vi "FPGA_encoder.vi"(3 "Encoder Channel B":refnum<k21>="ConnectorB/DIO1", 4 "Encoder Channel A":refnum<k21>="ConnectorB/DIO1", 5 "Velocity Interval (uSec)":u32=1000, 6 "Position Reset":bool) -> (0 "Velocity (Counts/Interval)":i32, 1 "Acceleration (Counts/Interval)":i32, 2 "Position (Counts)":i32)   [LabVIEW 2019]
doc: "This is an FPGA vi for Quadrature Encoder Velocity and Acceleration Estimation using CompactRIO. It requires as inputs a Fixed Time Interval for velocity and acceleration estimation.\n\nThis application is designed to work with an R-Series expansion setup using PCI/PXI-7811R FPGA device and a CompactRIO cRIO-9411 digital input module installed in slot 1 of the expansion chassis."
uses:
  <vilib>/rvi/Emulation/niFpgaGetClockAttributes.vi
  <vilib>/rvi/Emulation/niFpgaSctlEmulationGetInTimedLoop.vi
  <vilib>/rvi/Emulation/niFpgaEmulationReportErrorSimple.vi
  <vilib>/rvi/eio/common/nirviEmuTemplateMethod_errors.vi
  <vilib>/rvi/Emulation/niFpgaCriticalErrorInLSC.vi
  <vilib>/eio/EIONode/EIONode.xnode
  <vilib>/rvi/Arithmetic/AddSubMult/XNode/nirviSatArithmetic.xnode
panel:
  # "FPGA Application for Quadrature Encoder Velocity and \nAcceleration Estimation using CompactRIO.\n\nThis application is designed to work with an R-Series expansion setup \nusing FPGA-7811R and a CompactRIO cRIO-9411 digital input module \ninstalled in slot 1 of the expansion chassis."
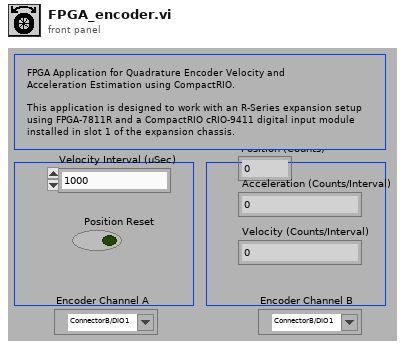
[diagram p1: front panel]
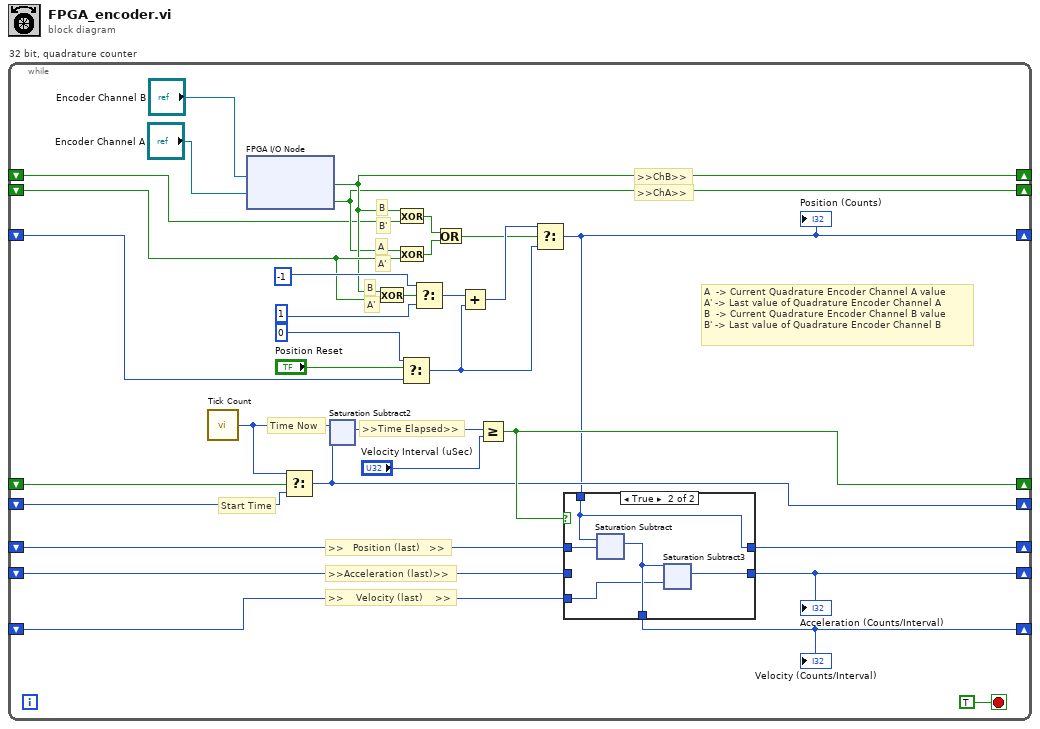
[diagram p0: block diagram]
diagram:
  n1 = while "32 bit, quadrature counter" {
    shift-right: [w22] -> _
    shift-left: _ -> [w8]
    shift-right: [w7] -> _
    shift-left: _ -> [w19]
    shift-right: [w21] -> _
    shift-left: _ -> [w23]
    shift-right: [w15] -> _
    shift-left: _ -> [w18]
    shift-right: [w10] -> _
    shift-left: _ -> [w16]
    shift-right: [w4] -> _
    shift-left: _ -> [w13]
    shift-right: [w5] -> _
    shift-left: _ -> [w12]
    shift-right: [w6] -> _
    shift-left: _ -> [w9]
    stop <- TRUE stop-if-true
    # "A  -> Current Quadrature Encoder Channel A value\nA' -> Last value of Quadrature Encoder Channel A\nB  -> Current Quadrature Encoder Channel B value\nB' -> Last value of Quadrature Encoder Channel B"
    # ">>Acceleration (last)>>"
    # "Start Time"
    # "A'"
    # "B"
    # "A'"
    # "A"
    # "B'"
    # "B"
    # ">>ChB>>"
    # ">>ChA>>"
    # ">>    Velocity (last)    >>"
    # ">>   Position (last)   >>"
    # "Time Now"
    # ">>Time Elapsed>>"
    n2 = call "Tick Count"() -> ("Tick Count(uSec)"=w11:u32)
    n3 = xnode "FPGA I/O Node"("FPGA I/O In"="Encoder Channel B", "FPGA I/O In"="Encoder Channel A") -> ("I/O Item"=w22:bool, "I/O Item"=w21:bool)  [unwired: 2 out]
    n4 = Select(t=w11, s=w18, f=w16) -> (s? t:f=w10:u32)
    n5 = xnode ("Saturation Subtract2")("x"=w11, "y"=w10) -> ("x-y"=w14:u32)
    n6 = Exclusive Or(1:w23, 2:w22) -> (0:w24:bool)
    n7 = Exclusive Or(1:w8, 2:w22) -> (0:w25:bool)
    n8 = Exclusive Or(1:w23, 2:w21) -> (0:w26:bool)
    n9 = Select(t=0 ("32 bit"), s="Position Reset", f=w19) -> (s? t:f=w31:i32)
    n10 = Select(t=-1 ("32 bit"), s=w24, f=1 ("32 bit")) -> (s? t:f=w29:i32)
    n11 = Or(x=w25, y=w26) -> (x .or. y?=w20:bool)
    n12 = Add(x=w29, y=w31) -> (x+y=w33:i32)
    n13 = Greater Or Equal?(x=w14, y="Velocity Interval (uSec)") -> (x >= y?=w15:bool)
    n14 = Select(t=w33, s=w20, f=w31) -> (s? t:f=w7:i32)
    "Position (Counts)" <- w7
    n15 = case shown="True" w15 {
      tunnel: w7 -> [_ w47]
      tunnel: w13 -> [w44 w51]
      tunnel: [w46 w50] -> w5
      tunnel: w12 -> [w46 w49]
      tunnel: [w45 w48] -> w6
      tunnel: w9 -> [w45 _]
      tunnel: [w44 w47] -> w4
      frame False {
      }
      frame True {
        n16 = xnode ("Saturation Subtract")("x"=w47, "y"=w51) -> ("x-y"=w50:i32)
        n17 = xnode ("Saturation Subtract3")("x"=w50, "y"=w49) -> ("x-y"=w48:i32)
      }
    }
    "Acceleration (Counts/Interval)" <- w6
    "Velocity (Counts/Interval)" <- w5
  }
